vi "Update moving conditions.vi"(8 "error in (no error)":errorcluster, 9 "Current position":cluster{"M1 pos":dbl, "M2 pos ":dbl}, 10 "Zero position":cluster{"M1":dbl, "M2":dbl}, 11 "Position params":T1) -> (0 "error out":errorcluster, 2 "Position reached?":bool[](array[boolean]), 3 "Position params out":T1)   [LabVIEW 2020]
doc: "Performs a check on the current position against the desired position. If the difference is within a certain range, the motor is set to IDLE status. A boolean array is returned to indicate whether or not each motor has reached its final position."
uses:
  controls/Motor direction ---typedef.ctl
  controls/Position arguments ---typedef.ctl
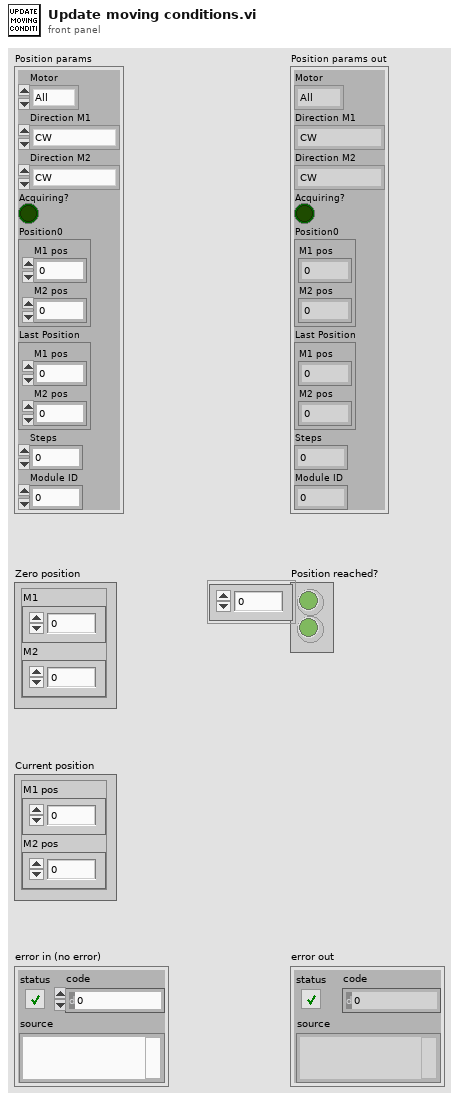
[diagram p1: front panel]
types:
  T1 = typedef "Position arguments ---typedef.ctl" = cluster{"Motor":enum16{"All", "M1", "M2"}, "Direction M1":T2, "Direction M2":T2, "Acquiring?":bool, "Position0":cluster{"M1 pos":dbl, "M2 pos ":dbl}, "Last Position":cluster{"M1 pos":dbl, "M2 pos ":dbl}, "Steps":i32, "Module ID":i32}
  T2 = typedef "Motor direction ---typedef.ctl" = enum16{"CW", "CCW", "IDLE"}
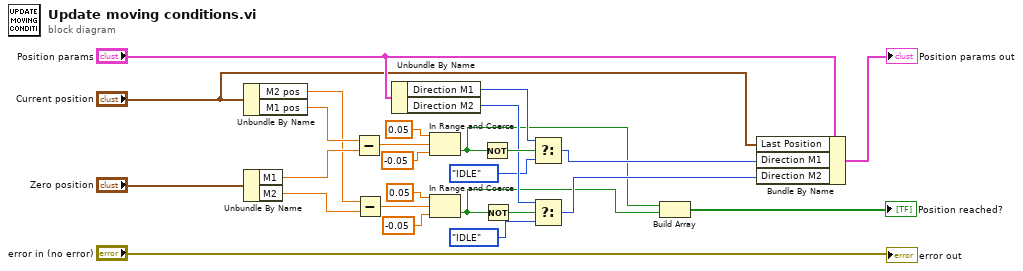
[diagram p0: block diagram]
diagram:
  n1 = Unbundle By Name("Current position") -> ("M2 pos"=w2:dbl, "M1 pos"=w3:dbl)
  n2 = Unbundle By Name("Zero position") -> ("M1"=w25:dbl, "M2"=w24:dbl)
  n3 = Subtract(x=w3, y=w25) -> (x-y=w23:dbl)
  n4 = Subtract(x=w2, y=w24) -> (x-y=w22:dbl)
  n5 = Unbundle By Name("Position params") -> ("Direction M1"=w14:T2, "Direction M2"=w13:T2)
  n6 = In Range and Coerce(upper limit=0.05, x=w23, lower limit=-0.05) -> (In Range?=w6:bool)  [unwired: 1 out]
  n7 = In Range and Coerce(upper limit=0.05, x=w22, lower limit=-0.05) -> (In Range?=w5:bool)  [unwired: 1 out]
  n8 = Not(x=w6) -> (.not. x?=w16:bool)
  n9 = Not(x=w5) -> (.not. x?=w15:bool)
  n10 = Select(t=w14, s=w16, f=Motor_direction_---typedef."IDLE") -> (s? t:f=w9:T2)
  n11 = Select(t=w13, s=w15, f=Motor_direction_---typedef."IDLE") -> (s? t:f=w8:T2)
  n12 = Build Array(w6, w5) -> (→"Position reached?":bool[])
  n13 = Bundle By Name(cluster="Position params", "Last Position"="Current position", "Direction M1"=w9, "Direction M2"=w8) -> (→"Position params out":T1)
  "error out" <- "error in (no error)"
